vi "Constants.vi"() -> ()   [LabVIEW 2020, in "AIM MIL-STD-1553 Scripting.lvlib"]
doc: "Use this Global VI to access the GUIDs assigned to the page resources of the Custom Device."
uses:
  AIM MIL-STD-1553 Scripting.lvlib
panel:
  in  "Tab Control":T1(tab)
  in  "GUID.Direction":string="FA190BB6-A886-4D21-B6CE-80C0AB8E079B"
  in  "GUID.Execution Monitor Section":string="88D6B64E-8237-4D92-B6F9-A951DB72295C"
  in  "GUID.Bus Status Load Channel":string="6266D492-4663-4381-8EC5-56E8335C0F3C"
  in  "GUID.Disabled Custom Device":string="652A4DB4-58F0-4BDA-95A2-9D3575DCD437"
  in  "GUID.Terminal Status Word":string="FA190BB6-A886-4D21-B6CE-80C0AB8E079B"
  in  "GUID.Logging":string="4CB50BEB-8E6A-4546-8042-31B06CA15D92"
  in  "GUID.Bus Status Count Channel":string="FC4AD462-4A88-4F50-B000-BF5D503E9DF7"
  in  "GUID.Command Channel":string="48F3F7DC-E070-4BBC-8C4E-16148CE3ABED"
  in  "GUID.Acyclic Frames":string="F3618C32-A245-4B8A-914D-0D9E1138716E"
  in  "GUID.Timestamp Channel":string="9D586491-763E-487A-BBEE-45C3FF68028A"
  in  "GUID.Bus Status Section":string="B1121469-E77C-4A90-A1D2-9B84A7A73F76"
  in  "GUID.Trigger Channel":string="F72813BC-5DD4-4A12-98AF-AF2ACE05D3F3"
  in  "GUID.Message":string="941EF121-AA5F-4AD9-93DB-CAE27E79D660"
  in  "GUID.Subaddress":string="2426566F-3E8E-40D3-A563-51778DC75F65"
  in  "GUID.Remote Terminal":string="DAD7DF52-76CE-4065-A310-4B0BE1A080E9"
  in  "GUID.Bus Controller":string="21F44F0E-FD4D-4419-B4D7-B1E61B610078"
  in  "GUID.Configuration Files":string="4CECF82F-8008-49E9-B19E-08BF1610E0CB"
  in  "GUID.Channel":string="FC881C7F-B684-4A91-BDA4-2949993470AC"
  in  "GUID.Port":string="4AC0C534-27A2-477F-ADF0-74A57AB22AEF"
  in  "GUID.Custom Device":string="CA7BC298-6196-4AAD-B3DA-33017CCDCA53"
  in  "Execution Monitor Section":string="Execution Monitor"
  in  "Bus Status Section":string="Bus Status"
  in  "Remote Terminal Name":string="Remote Terminal Name"
  in  "Logging":string="Logging"
  in  "Scale Offset":string="Scale Offset"
  in  "Scale Multiplier":string="Scale Multiplier"
  in  "Signed":string="Signed"
  in  "Encoding":string="Encoding"
  in  "Size in Bits":string="Size in Bits"
  in  "Start Index":string="Start Index"
  in  "Unit":string="Unit"
  in  "Default Value":string="Default Value"
  in  "Create Timestamp Channel":string="Create Timestamp Channel"
  in  "Number of Words":string="Number of Words"
  in  "Tx Subaddress":string="Tx Subaddress"
  in  "Tx Terminal Address":string="Tx Terminal Address"
  in  "Rx Subaddress":string="Rx Subaddress"
  in  "Rx Terminal Address":string="Rx Terminal Address"
  in  "Message Type":string="Message Type"
  in  "Parameter":string="Parameter"
  in  "Message":string="Message"
  in  "Mode Code":string="Mode Code"
  in  "Acyclic Frame":string="Acyclic Frame"
  in  "Subaddress":string="Subaddress"
  in  "Custom Device":string="AIM MIL-STD-1553"
  in  "Global Error Count":string="Global Error Count"
  in  "Secondary Bus Average Load (%)":string="Secondary Bus Average Load (%)"
  in  "Secondary Bus Current Load (%)":string="Secondary Bus Current Load (%)"
  in  "Primary Bus Average Load (%)":string="Primary Bus Average Load (%)"
  in  "Primary Bus Current Load (%)":string="Primary Bus Current Load (%)"
  in  "Global Message Count":string="Global Message Count"
  in  "PXI Slot Number":string="PXI Slot Number"
  in  "Card Number":string="Card Number"
  in  "Acyclic Frames":string="Acyclic Frames"
  in  "Timestamp":string="Timestamp"
  in  "Trigger":string="Trigger"
  in  "Status":string="Status"
  in  "Remote Terminal":string="Remote Terminal"
  in  "Stop":string="Stop"
  in  "Start":string="Start"
  in  "Bus Controller":string="Bus Controller"
  in  "Configuration Files":string="Configuration Files"
  in  "Channel":string="Channel"
  in  "Port":string="Port"
  in  "Prop.Rx.Async":string="Run Rx Asynchronously"
  in  "Prop.Timing.Mode":string="timing mode"
  in  "Prop.Execution Time.Logging":string="Logging Execution Unit Time"
  in  "Prop.Execution Time.Tx":string="Tx Execution Unit Time"
  in  "Prop.Execution Time.Triggers":string="Triggers Execution Unit Time"
  in  "Prop.Execution Time.Rx":string="Rx Execution Unit Time"
  in  "Prop.Starting.Buffer.Index":string="Starting Buffer Index"
  in  "Prop.Protocol.MinorFrames.Period":string="Minor Frame Period"
  in  "Prop.Trigger.AcyclicFrame.%s.Messages":string="Acyclic Frame.%s.Messages"
  in  "Prop.Coupling.Mode":string="coupling mode"
  in  "Prop.Bus.Selection":string="bus selection"
  in  "Prop.Protocol.MinorFrames.%s.Messages":string="Minor Frames.%s.Messages"
  in  "Prop.Protocol.MinorFrames":string="Minor Frames"
  in  "Prop.Protocol.MajorFrames.%s.MinorFrames":string="Major Frames.%s.Minor Frames"
  in  "Prop.Protocol.MajorFrames":string="Major Frames"
  in  "Prop.Logging.File Name Timestamp":string="File Name Timestamp"
  in  "Prop.Logging.File":string="File"
  in  "Prop.Logging.Data Word Format":string="Data Word Format"
  in  "Prop.Logging.Enabled":string="Enabled"
  in  "Prop.Logging.Directory":string="Log Directory"
  in  "Prop.Parameters.File.Required":string="Parameters File Required"
  in  "Prop.Mode.Code":string="modeCode"
  in  "Prop.Message.Type":string="messageType"
  in  "Prop.Direction":string="direction"
  in  "Prop.Trigger.AcyclicFrame":string="Acyclic Frame"
  in  "Prop.Message.Name":string="messageName"
  in  "Prop.Number.Of.Words":string="numberOfWords"
  in  "Prop.Parameter":string="parameter"
  in  "Prop.Unit":string="unit"
  in  "Prop.Offset":string="offset"
  in  "Prop.Scale":string="scale"
  in  "Prop.Signed":string="signed"
  in  "Prop.Encoding":string="encoding"
  in  "Prop.SizeInBits":string="numberOfBits"
  in  "Prop.StartIndex":string="startBit"
  in  "Prop.DefaultValue":string="defaultValue"
  in  "Prop.Name":string="name"
  in  "Prop.Subaddress":string="subAddress"
  in  "Prop.Terminal.Address":string="terminalAddress"
  in  "Prop.Parameters.File":string="Win Parameters File Path"
  in  "Prop.Hardware.Configuration.File":string="Hardware Configuration File"
  in  "Prop.PXI.Slot.Number":string="PXI Slot Number"
  in  "Prop.Initialization.Method":string="Initialization Method"
  in  "Prop.BIU.Number":string="biu number"
  in  "Prop.Card.Number":string="card number"
  in  "Compiled.Settings":string="Compiled.Settings"
  in  "Error Parameters Configuration File MD5":string="error_key_MIL-STD-1553_parameters_cfg_file_MD5"
  in  "Error Parameters Configuration File":string="error_key_MIL-STD-1553_parameters_cfg_file"
  in  "Error Hardware Configuration File":string="error_key_MIL-STD-1553_hardware_cfg_file"
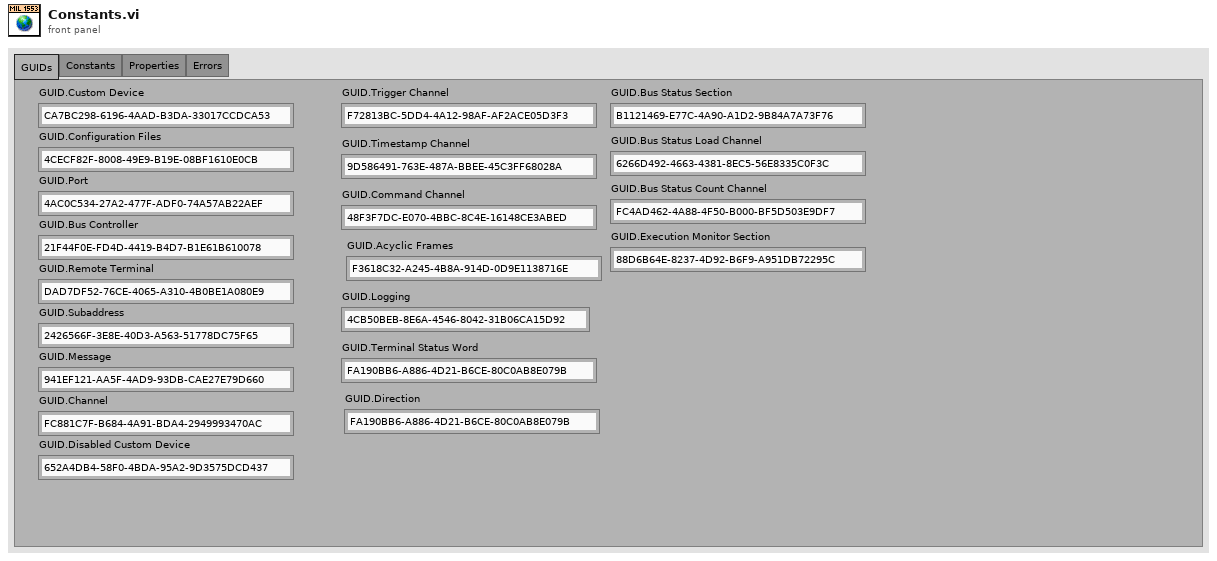
[diagram p1: front panel]
types:
  T1 = enum32{"GUIDs", "Constants", "Properties", "Errors"}
diagram:
